vi "GetLoadedProgram.vi"(0 "Universal Robot.lvclass in":refnum<class "Universal Robot.lvclass">, 5 "error in (no error)":errorcluster) -> (14 "Universal Robot.lvclass out":refnum<class "Universal Robot.lvclass">, 15 "loaded program":string, 19 "error out":errorcluster)   [LabVIEW 2019, in "Universal Robot.lvclass"]
uses:
  Universal Robot.lvclass
  Universal Robot.lvclass/Universal Robot.ctl
  Client Interfaces/Dashboard Server/Dashboard Server.lvclass
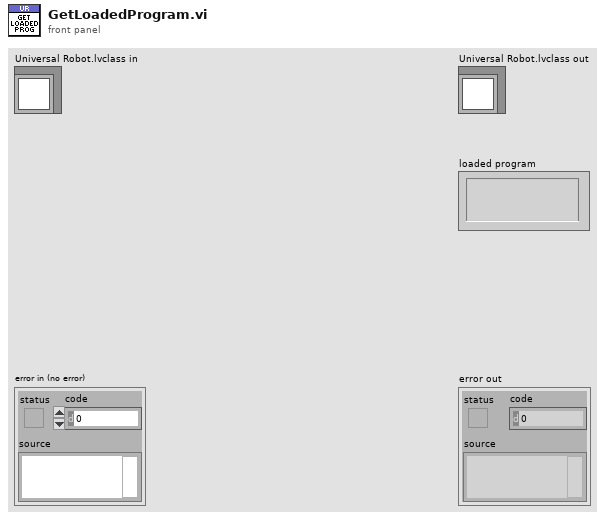
[diagram p1: front panel]
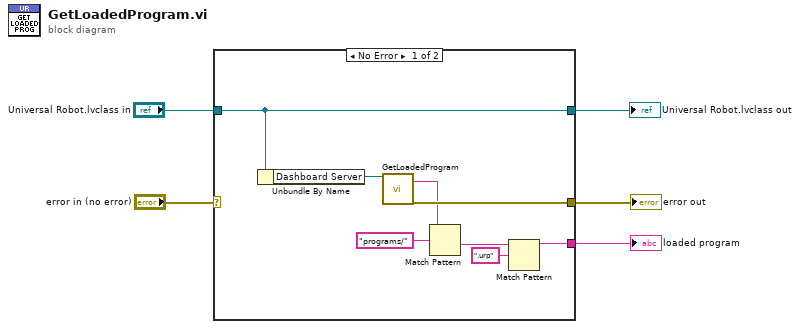
[diagram p0: block diagram]
diagram:
  n1 = case shown="No Error" "error in (no error)" {
    selector: "error in (no error)" -> [_ w15]
    tunnel: [w11 w15] -> w4
    tunnel: "Universal Robot.lvclass in" -> [w13 w14]
    tunnel: [w13 w14] -> w2
    tunnel: [w6 _] -> w1
    frame No Error {
      n2 = Unbundle By Name(w13) -> ("Dashboard Server"=w12:refnum<class "Dashboard Server.lvclass">)
      n3 = call-dynamic "GetLoadedProgram.vi"("DashboardServer in"=w12) -> ("loadedProgram"=w7:string, "error out"=w11:errorcluster)  [unwired: 16 in, 1 out]
      n4 = Match Pattern(string=w7, regular expression="programs/") -> (after substring=w9:string)  [unwired: 1 in, 3 out]
      n5 = Match Pattern(string=w9, regular expression=".urp") -> (before substring=w6:string)  [unwired: 1 in, 3 out]
    }
    frame Error {
    }
  }
  "error out" <- w4
  "Universal Robot.lvclass out" <- w2
  "loaded program" <- w1
